vi "Read Measurement.vi"(8 "error in (no error)":errorcluster, 10 "Vin SMU Channel":string, 11 "IVI Refnum in":refnum<k15>) -> (0 "error out":errorcluster, 2 "Current":dbl, 3 "Voltage":dbl)   [LabVIEW 2021, in "SMU_Voltage Measurement.lvlib"]
uses:
  SMU_Voltage Measurement.lvlib
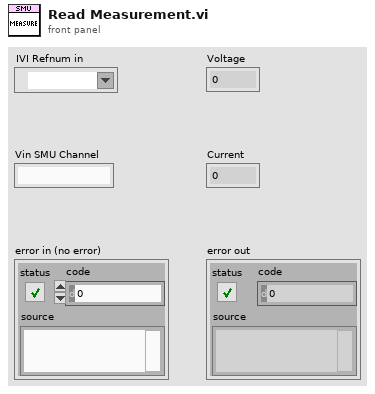
[diagram p1: front panel]
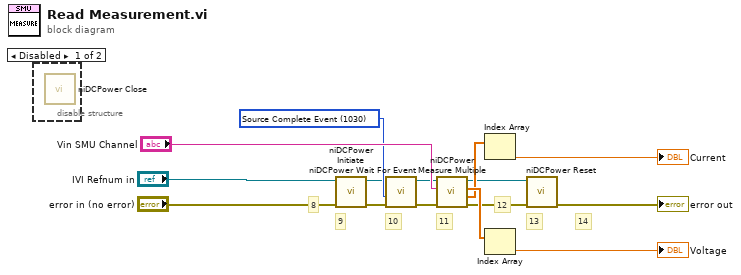
[diagram p0: block diagram]
diagram:
  w7 = 1030 items=["Source Complete Event"=1030, "Measure Complete Event"=1031, "Sequence Iteration Complete Event"=1032, "Sequence Engine Done Event"=1033] ("event")
  # "14"
  # "9"
  # "11"
  # "10"
  # "12"
  # "13"
  # "8"
  n1 = disable-structure shown="Disabled" {
    frame Disabled {
      n2 = call <instrlib>:"niDCPower Close.vi"() -> ()  [unwired: 11 in, 1 out]
    }
    frame Enabled {
    }
  }
  n3 = call <instrlib>:"niDCPower Initiate.vi"("error in (no error)"="error in (no error)", "instrument handle"="IVI Refnum in") -> ("error out"=w5:errorcluster, "instrument handle out"=w3:refnum<k15>)  [unwired: 2 in, 6 out]
  n4 = call <instrlib>:"niDCPower Wait For Event.vi"("error in (no error)"=w5, "event"=w7, "instrument handle"=w3) -> ("error out"=w6:errorcluster, "instrument handle out"=w4:refnum<k15>)  [unwired: 1 in, 6 out]
  n5 = call <instrlib>:"niDCPower Measure Multiple.vi"("error in (no error)"=w6, "channel name"="Vin SMU Channel", "instrument handle"=w4) -> ("error out"=w2:errorcluster, "current measurements"=w8:dbl[], "voltage measurements"=w9:dbl[], "instrument handle out"=w1:refnum<k15>)  [unwired: 5 out]
  n6 = Index Array(array=w8) -> (element=→"Current":dbl)  [unwired: 1 in]
  n7 = Index Array(array=w9) -> (element=→"Voltage":dbl)  [unwired: 1 in]
  n8 = call <instrlib>:"niDCPower Reset.vi"("error in (no error)"=w2, "instrument handle"=w1) -> ("error out"=→"error out":errorcluster)  [unwired: 2 in, 7 out]
